vi "dfd_FFT Spectrum to FRF.vi"(4 "phase view":T1, 7 "use half band?":bool=TRUE, 8 "error in (no error)":errorcluster, 9 "magnitude":u16(ring)=1 items=["Linear", "dB", "Zero phase"], 11 "FFT {X}":cdb[](array[numeric]) format="%.2f") -> (0 "error out":errorcluster, 2 "phase":dbl[](array[numeric]) format="%.2f", 3 "amplitude":dbl[](array[numeric]) format="%.2f")   [LabVIEW 2017, in "NI_DigFilterLicensed.lvlib"]
uses:
  <vilib>/addons/Digital Filter Design/NI_DigFilterLicensed.lvlib
  <vilib>/addons/Digital Filter Design/_Objects.llb/DFD Phase Setting.ctl
  <vilib>/Analysis/NI_AALPro.lvlib
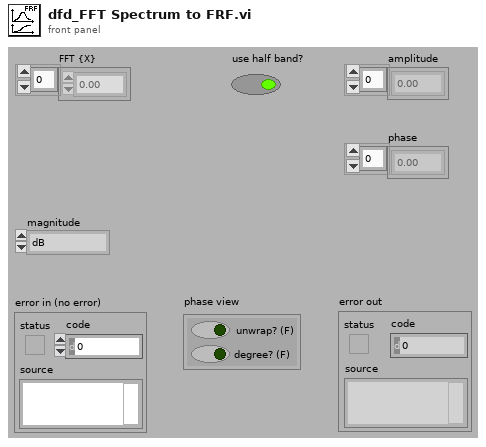
[diagram p1: front panel]
types:
  T1 = typedef "NI_DigFilterLicensed.lvlib/DFD Phase Setting.ctl" = cluster{"unwrap? (F)":bool, "degree? (F)":bool}
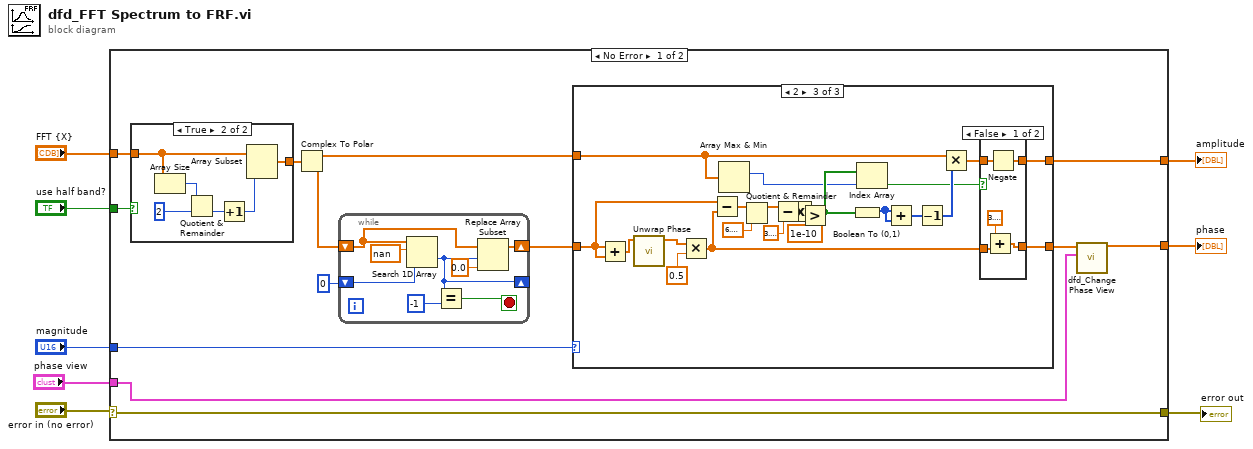
[diagram p0: block diagram]
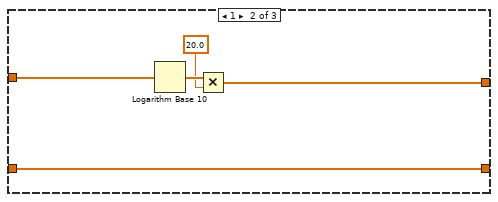
[diagram p3: hidden frame]
diagram:
  n1 = case shown="No Error" "error in (no error)" {
    selector: "error in (no error)" -> [w16 w73]
    tunnel: [w21 _] -> w8
    tunnel: [w10 _] -> w7
    tunnel: "phase view" -> [w9 _]
    tunnel: "FFT {X}" -> [w20 _]
    tunnel: [w16 w73] -> w3
    tunnel: "use half band?" -> [w15 _]
    tunnel: "magnitude" -> [w12 _]
    frame No Error {
      n2 = case shown="True" w15 {
        tunnel: w20 -> [w66 w68]
        tunnel: [w66 w67] -> w19
        frame False {
        }
        frame True {
          n3 = Array Size(array=w68) -> (size(s)=w72:i32)
          n4 = Quotient & Remainder(x=w72, y=2) -> (floor(x/y)=w70:i32)  [unwired: 1 out]
          n5 = Increment(x=w70) -> (x+1=w69:i32)
          n6 = Array Subset(array=w68, length=w69) -> (w67:cdb[])  [unwired: 1 in]
        }
      }
      n7 = Complex To Polar(r * e^(i*theta)=w19) -> (r=w18:dbl[], theta=w17:dbl[])
      n8 = while {
        shift-right: [w60] -> _
        shift-left: 0 ("index of element") -> [w58]
        shift-right: [w61] -> w13
        shift-left: w17 -> [w64]
        stop <- w62 stop-if-true
        n9 = Search 1D Array(1D array=w64, element=nan, start index (0)=w58) -> (index of element=w60:i32)
        n10 = Equal?(x=w60, y=-1) -> (x = y?=w62:bool)
        n11 = Replace Array Subset(array=w64, new element=0.0 ("new element/subarray"), index=w60) -> (w61:dbl[])
      }
      n12 = case shown="2" w12 {
        tunnel: [w23 w25 w50] -> w21
        tunnel: [w22 w24 w49] -> w11
        tunnel: w18 -> [w23 w26 w48]
        tunnel: w13 -> [w22 w24 w29]
        frame 0, Default {
        }
        frame 1 {
          n13 = Logarithm Base 10(1:w26) -> (0:w28:dbl[])
          n14 = Multiply(x=w28, y=20.0) -> (x*y=w25:dbl[])
        }
        frame 2 {
          n15 = Add(x=w29, y=w29) -> (x+y=w47:dbl[])
          n16 = call <vilib>:"Unwrap Phase.vi"("Phase"=w47) -> ("Unwrapped Phase"=w46:dbl[])  [unwired: 1 in, 9 out]
          n17 = Multiply(x=w46, y=0.5) -> (x*y=w34:dbl[])
          n18 = Subtract(x=w29, y=w34) -> (x-y=w44:dbl[])
          n19 = Array Max & Min(array=w48) -> (max index (indices)=w37:i32)  [unwired: 3 out]
          n20 = Quotient & Remainder(x=w44, y=6.283185307179586) -> (x-y*floor(x/y)=w32:dbl[])  [unwired: 1 out]
          n21 = Subtract(x=w32, y=3.141592653589793) -> (x-y=w33:dbl[])
          n22 = Absolute Value(x=w33) -> (abs(x)=w30:dbl[])
          n23 = Greater?(x=w30, y=1e-10) -> (0:w38:bool[])
          n24 = Boolean To (0,1)(Boolean=w38) -> (0, 1=w41:i16[])
          n25 = Index Array(array=w38, index=w37) -> (element=w36:bool)
          n26 = Add(x=w41, y=w41) -> (x+y=w40:i16[])
          n27 = Decrement(x=w40) -> (x-1=w39:i16[])
          n28 = Multiply(x=w48, y=w39) -> (x*y=w35:dbl[])
          n29 = case shown="False" w36 {
            tunnel: w35 -> [w55 w57]
            tunnel: [w54 w57] -> w50
            tunnel: w34 -> [w53 w56]
            tunnel: [w51 w56] -> w49
            frame False {
              n30 = Add(x=3.141592653589793, y=w53) -> (x+y=w51:dbl[])
              n31 = Negate(x=w55) -> (-x=w54:dbl[])
            }
            frame True {
            }
          }
        }
      }
      n32 = call <vilib>:"dfd_Change Phase View.vi"("phase view"=w9, "phase in (rad)"=w11) -> ("phase out"=w10:dbl[])  [unwired: 9 out]
    }
    frame Error {
    }
  }
  "amplitude" <- w8
  "phase" <- w7
  "error out" <- w3
